vi "DUT_Query.vi"(4 "error in (no error)":errorcluster, 6 "command":string, 7 "connection ID":refnum<k5>) -> (3 "error out":errorcluster, 5 "reply":string, 8 "elapsed ms":dbl, 11 "connection ID out":refnum<k5>)   [LabVIEW 2026]
doc: "Sends one command to the DUT over an already-open TCP connection,\nreturns the trimmed reply and the round-trip time in ms, and appends\none row to data\\trace.csv. The caller owns the connection: it is\npassed in and handed back out."
uses:
  <vilib>/Utility/error.llb/Trim Whitespace (string).vi
  <vilib>/Utility/error.llb/Trim Whitespace One-Sided.vi
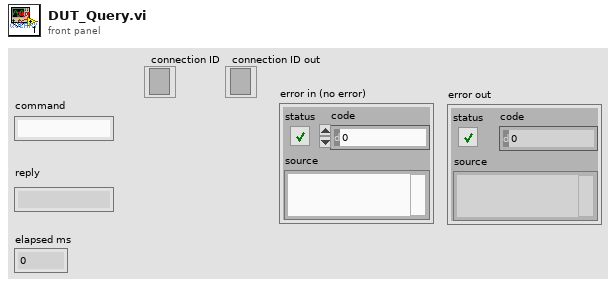
[diagram p1: front panel]
types:
  T1 = enum16{"open", "replace", "create", "open or create", "replace or create", "replace or create with confirmation"}
  T2 = enum16{"Standard", "Buffered", "CRLF", "Immediate"}
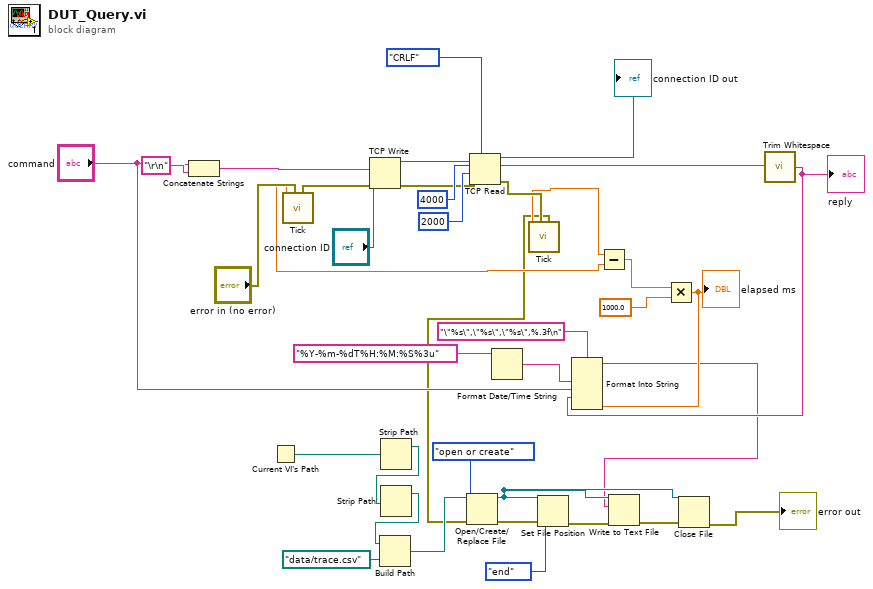
[diagram p0: block diagram]
diagram:
  n1 = Concatenate Strings "Concatenate Strings"("command", "\r\n" ("string")) -> (w37:string)
  n2 = Current VI's Path() -> (path=w14:path)
  n3 = call "Tick.vi"("error in (no error)"="error in (no error)") -> ("error out"=w27:errorcluster, "seconds"=w23:dbl)  [unwired: 9 in]
  n4 = TCP Write(connection ID="connection ID", data in=w37, error in (no error)=w27) -> (connection ID out=w31:refnum<k5>, error out=w30:errorcluster)  [unwired: 1 in, 1 out]
  n5 = Strip Path(path=w14) -> (stripped path=w13:path)  [unwired: 1 out]
  n6 = Strip Path(path=w13) -> (stripped path=w12:path)  [unwired: 1 out]
  n7 = Build Path(base path=w12, name or relative path=path "data/trace.csv") -> (appended path=w10:path)
  n8 = TCP Read(connection ID=w31, bytes to read=4000, error in (no error)=w30, 7:T2."CRLF" ("mode (standard)"), 9:2000 ("timeout ms (25000)")) -> (connection ID out=→"connection ID out":refnum<k5>, data out=w29:string, error out=w25:errorcluster)
  n9 = Format Date/Time String(time format string (%c)="%Y-%m-%dT%H:%M:%S%3u") -> (date/time string=w18:string)  [unwired: 2 in]
  n10 = call "Tick.vi"("error in (no error)"=w25) -> ("error out"=w2:errorcluster, "seconds"=w24:dbl)  [unwired: 9 in]
  n11 = Open/Create/Replace File(file path (use dialog)=w10, error in=w2, operation (0:open)=T1."open or create") -> (refnum out=w7:refnum<file>, error out=w6:errorcluster)  [unwired: 3 in, 1 out]
  n12 = Set File Position(refnum=w7, from (0:start)=enum16{"start", "end", "current"}."end", error in=w6) -> (error out=w5:errorcluster)  [unwired: 1 in, 1 out]
  n13 = Subtract(x=w24, y=w23) -> (x-y=w22:dbl)
  n14 = Multiply(x=w22, y=1000.0) -> (x*y=w15:dbl)
  "elapsed ms" <- w15
  n15 = call-poly <vilib>:"Trim Whitespace.vi"("string"=w29) -> ("trimmed string"=w16:string)  [unwired: 1 in]
  "reply" <- w16
  n16 = Format Into String(format string="\"%s\",\"%s\",\"%s\",%.3f\n", w18, "command", w16, w15) -> (resulting string=w3:string)  [unwired: 2 in, 1 out]
  n17 = Write to Text File(file (use dialog)=w7, text=w3, error in=w5) -> (error out=w4:errorcluster)  [unwired: 1 in, 2 out]
  n18 = Close File(refnum=w7, error in=w4) -> (error out=→"error out":errorcluster)  [unwired: 1 out]
